vi "mqttCmdCreate.vi"(8 "error in (no error)":errorcluster, 10 "mqtt instance":refnum<class "MQTT Client.lvclass">) -> (0 "error out":errorcluster, 3 "mqttCmdPing out":refnum<class "PingMqttMsg.lvclass">)   [LabVIEW 2020, in "PingMqttMsg.lvclass"]
uses:
  PingMqttMsg.lvclass
  MQTT Client.lvclass
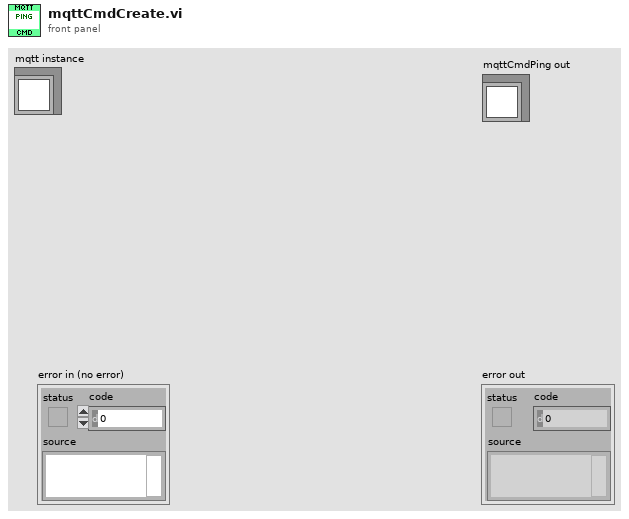
[diagram p1: front panel]
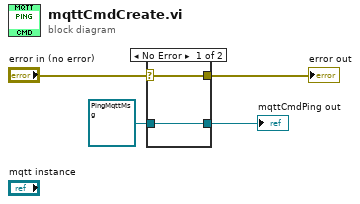
[diagram p0: block diagram]
diagram:
  n1 = case shown="No Error" "error in (no error)" {
    selector: "error in (no error)" -> [w6 w8]
    tunnel: [w6 w8] -> w3
    tunnel: [w5 w7] -> w1
    tunnel: refnum<class "PingMqttMsg.lvclass"> refnum ("mqttCmdPing in") -> [w5 w7]
    frame No Error {
    }
    frame Error {
    }
  }
  "error out" <- w3
  "mqttCmdPing out" <- w1
